vi "周期设置_多参数.vi"() -> ()   [LabVIEW 2016, in "斯坦道原位多参数.lvlib"]
uses:
  <vilib>/Utility/miscctls.llb/LVPointTypeDef.ctl
panel:
  in  "运行周期":T1
  # "运行模式："
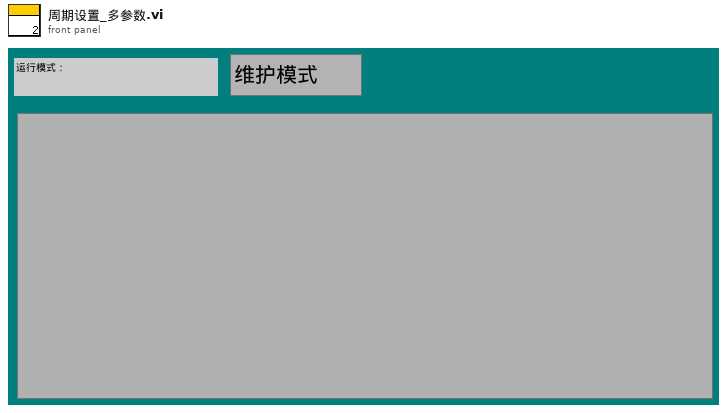
[diagram p1: front panel]
types:
  T1 = cluster{"运行模式":enum16{"维护模式", "常规模式", "应急模式", "质控模式"}, "24H周期设置":bool[]}
  T2 = typedef "LVPointTypeDef.ctl" = cluster{"Horizontal":i16, "Vertical":i16}
  T3 = typedef "斯坦道原位多参数.lvlib/水样测试启动自定义输入参数.ctl" = cluster{"测量模式":string, "数据类型":string}
  T4 = typedef "LVDateTimeRec.ctl" = cluster{"秒数的小数部分":dbl, "秒":i32, "分":i32, "时":i32, "日":i32, "月":i32, "年":i32, "天数（周）":i32, "天数（年）":i32, "DST":i32}
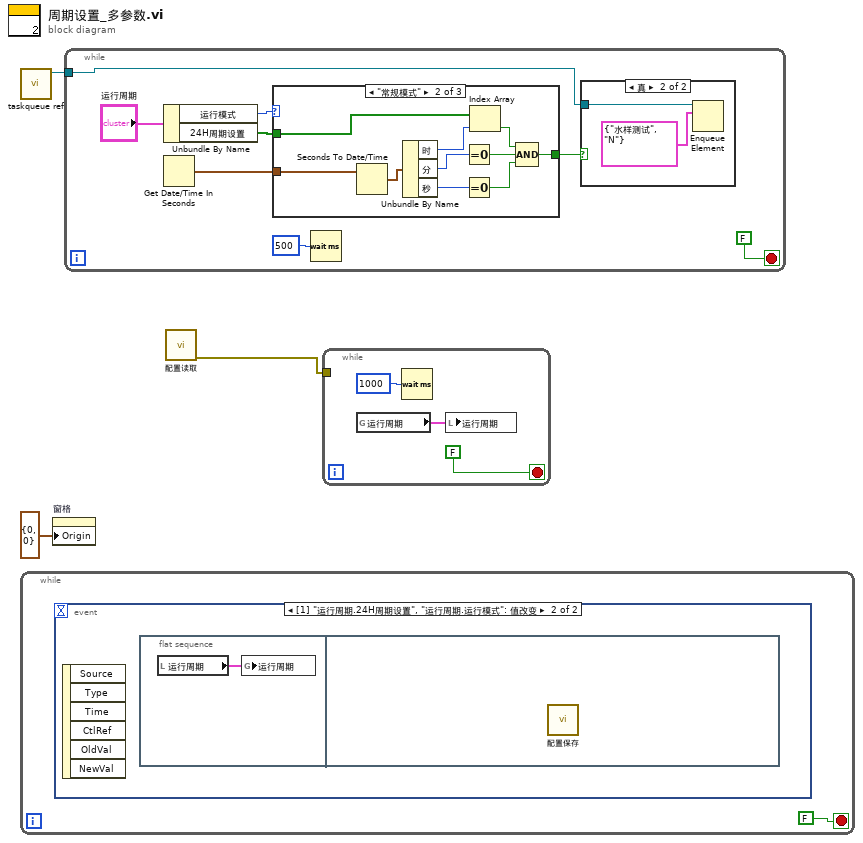
[diagram p0: block diagram]
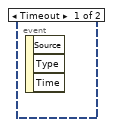
[diagram p2: hidden frame]
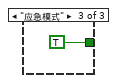
[diagram p5: hidden frame]
diagram:
  n1 = call "taskqueue ref.vi"() -> ("队列输出"=w1:refnum<queue>)  [unwired: 10 in, 1 out]
  n2 = while {
    stop <- FALSE stop-if-true
    n3 = event shown="[1] \"运行周期.24H周期设置\", \"运行周期.运行模式\": 值改变" {
      selector: _ -> [_ _]
      dyn-events: _ -> [_ _]
      timeout: _ -> [_ _]
      event Timeout {
        n4 = event-data() -> ()  [unwired: 1 in, 3 out]
      }
      event "运行周期.24H周期设置", "运行周期.运行模式": Value Change {
        n5 = event-data() -> ()  [unwired: 1 in, 6 out]
        n6 = flat-sequence {
          frame #0 {
            n7 = local read "运行周期"() -> (w5:T1)
            n8 = global write "多参数断电保存全局变量.vi" "运行周期"(w5) -> ()
          }
          frame #1 {
            n9 = call "配置保存.vi"() -> ()  [unwired: 11 in, 1 out]
          }
        }
      }
    }
  }
  n10 = property on="窗格" class="Pane"("Origin"=T2 {"Horizontal"=0, "Vertical"=0} ("原点")) -> ()  [unwired: 2 in, 2 out]
  n11 = while {
    tunnel: w1 -> [w6]
    stop <- FALSE stop-if-true
    n12 = Unbundle By Name("运行周期") -> ("运行模式"=w7:enum16{"维护模式", "常规模式", "应急模式", "质控模式"}, "24H周期设置"=w9:bool[])
    n13 = Get Date/Time In Seconds() -> (seconds since 1Jan1904=w13:timestamp)
    n14 = case shown="\"常规模式\"" w7 {
      tunnel: w13 -> [_ w25 _]
      tunnel: w9 -> [_ w22 _]
      tunnel: [_ w16 TRUE] -> w8
      frame "维护模式", Default {
      }
      frame "常规模式" {
        n15 = Seconds To Date/Time(time stamp (now)=w25) -> (date time rec=w24:T4)  [unwired: 1 in]
        n16 = Unbundle By Name(w24) -> ("时"=w23:i32, "分"=w21:i32, "秒"=w20:i32)
        n17 = Equal To 0?(x=w21) -> (x = 0?=w18:bool)
        n18 = Equal To 0?(x=w20) -> (x = 0?=w17:bool)
        n19 = Index Array(array=w22, index=w23) -> (element=w19:bool)
        n20 = Compound Arithmetic op=AND ("复合运算")(w19, w18, w17) -> (w16:bool)
      }
      frame "应急模式" {
      }
    }
    n21 = Wait (ms)(milliseconds to wait=u32 500 ("等待时间（毫秒）")) -> ()  [unwired: 1 out]
    n22 = case shown="真" w8 {
      tunnel: w6 -> [_ w15]
      frame False {
      }
      frame True {
        n23 = Enqueue Element(queue=w15, element=T3 {"测量模式"="水样测试", "数据类型"="N"} ("启动参数")) -> ()  [unwired: 2 in, 3 out]
      }
    }
  }
  n24 = call "配置读取.vi"() -> ("error out"=w3:errorcluster)  [unwired: 11 in]
  n25 = while {
    tunnel: w3 -> [_]
    stop <- FALSE stop-if-true
    n26 = global read "多参数断电保存全局变量.vi" "运行周期"() -> (w27:T1)
    n27 = Wait (ms)(milliseconds to wait=u32 1000 ("等待时间（毫秒）")) -> ()  [unwired: 1 out]
    n28 = local write "运行周期"(w27) -> ()
  }
